vi "fpga_4w BufferControl.vi"(7 "DR":bool, 9 "RFI":bool, 12 "RFO":bool) -> (4 "buff enable":bool, 8 "output valid":bool, 10 "ready for input":bool, 14 "logic enable":bool)   [LabVIEW 2011, in "NI_EP_Resample_FPGA.lvlib"]
uses:
  <vilib>/addons/Electrical Power/PQ/Resampling/NI_EP_Resample_FPGA.lvlib
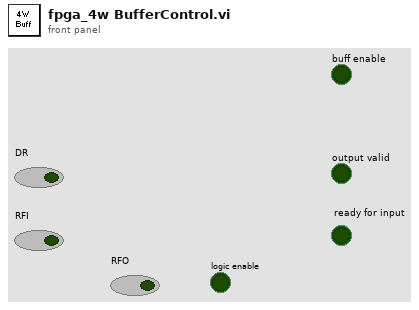
[diagram p1: front panel]
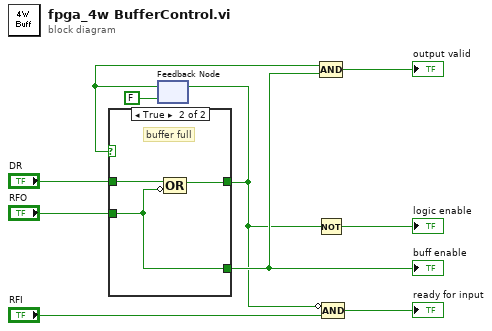
[diagram p0: block diagram]
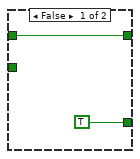
[diagram p2: hidden frame]
diagram:
  n1 = feedback #1(FALSE) -> (w2:bool)
  n2 = case shown="True" w2 {
    tunnel: "DR" -> [w11 w14]
    tunnel: "RFO" -> [_ w13]
    tunnel: [w11 w15] -> w4
    tunnel: [TRUE w13] -> w6
    frame False {
    }
    frame True {
      # "buffer full"
      n3 = Compound Arithmetic op=OR(w14, invert w13) -> (w15:bool)
    }
  }
  "buff enable" <- w6
  n4 = feedback-in #1(w4) -> ()
  n5 = Not(x=w4) -> (.not. x?=→"logic enable":bool)
  n6 = Compound Arithmetic op=AND(w2, w6) -> (→"output valid":bool)
  n7 = Compound Arithmetic op=AND(invert w4, "RFI") -> (→"ready for input":bool)
